vi "Dashboard Main.vi"() -> ()   [LabVIEW 2015]
uses:
  <vilib>/Utility/miscctls.llb/LVRowAndColumnTypeDef.ctl
  <vilib>/event_ctls.llb/eventvkey.ctl
  <vilib>/Rock Robotics/WPI/Dashboard/WPI_DashboardLogging Global.vi
  <vilib>/Rock Robotics/Network Tables/NT Read Boolean.vi
  <vilib>/Rock Robotics/Network Tables/NT Write Numeric Array.vi
  <vilib>/Utility/config.llb/Write Key (String).vi
  <vilib>/Utility/config.llb/Write Key (I32).vi
  <vilib>/Utility/config.llb/NI_LVConfig.lvlib
panel:
  in  "Low Bar":bool
  in  "Cheval":bool
  in  "Portcullis":bool
  in  "Moat":bool
  in  "Ramparts":bool
  in  "R. Terrain":bool
  in  "Rock Wall":bool
  in  "Spy":bool
  in  "Shoot":bool=TRUE
  in  "5":bool
  in  "4":bool
  in  "3":bool
  in  "2":bool
  in  "1":bool
  in  "TCP":refnum<k5>
  in  "Rec Mode":enum32{"Stop", "Record", "Playback"}(radio)
  in  "Vision":u16(ring) items=["Camera Off", "USB Camera SW", "USB Camera HW", "IP Camera"]
  out "Camera IP":string
  out "Image Message":string="Timeout in Camera Communications"
  in  "Dashboard Tab":T1(tab)
  out "Vision\nActive":bool
  out "Level":u8(slide) scale=0.0..3.0
  out "FIRE!!!!":bool
  out "Harvester":dbl
  out "Rotate":dbl
  out "Arm":dbl
  in  "Select Auto":string(combo)
  out "NT Connection":bool
  in  "Camera Settings":T2={"Frame Rate"=30, "Compression"=30, "Size"=1} {"Frame Rate" scale=1.0..30.0; "Size" items=["640x480", "320x240", "160x120"]}
  out "Mode":T3(ring)=enum."Auto Disabled"
  in  "DB Camera Config":bool
  out "fps":dbl format="%#.1g"
  out "Mbps":dbl format="%#.1g"
  out "Mbps LED":bool
  out "Shooter":dbl(knob) scale=0.0..1000.0
  out "Ball Detected":bool
  in  "Custom Auto":bool
  in  "Do Nothing":bool
  in  "File Path":path=path "C:/Users/Rick/Desktop/Robot-2016/autonomous.apple"
  in  "Automode":i32
  out "Error Log":string
  in  "Test Slider":dbl(slide) scale=0.0..100.0 scale format="%#_3g"
  in  "On/Off":bool caption="Solenoid"
  in  "Test Name":u16(ring) items=["Select the test to run..."]
  in  "Test Tree":string(tree)
  in  "Motor":cluster{"Value":dbl, "Enable":bool} {"Value" scale=-1.0..1.0 scale format="%#_3g"}
  out "Progress":T4 {"Test Progress" scale=0.0..100.0}
  in  "Rev/Fwd":cluster{"Forward":bool, "Reverse":bool}
  in  "Test Ring":u16(ring) items=["Monochrome", "Color"]
  out "Cmd Status":string
  in  "Execute Command":bool
  in  "Command Params":string[][](table)
  in  "Command Selection":i32(listbox)
  in  "CheckList":i32(listbox)
  out "Tree":string(tree)
  out "Camera Image":T5(plugin-control)
  out "Background":bool
  # "Batter Shot"
  # "Normal Shot"
  # "Transport"
  # "Harvest"
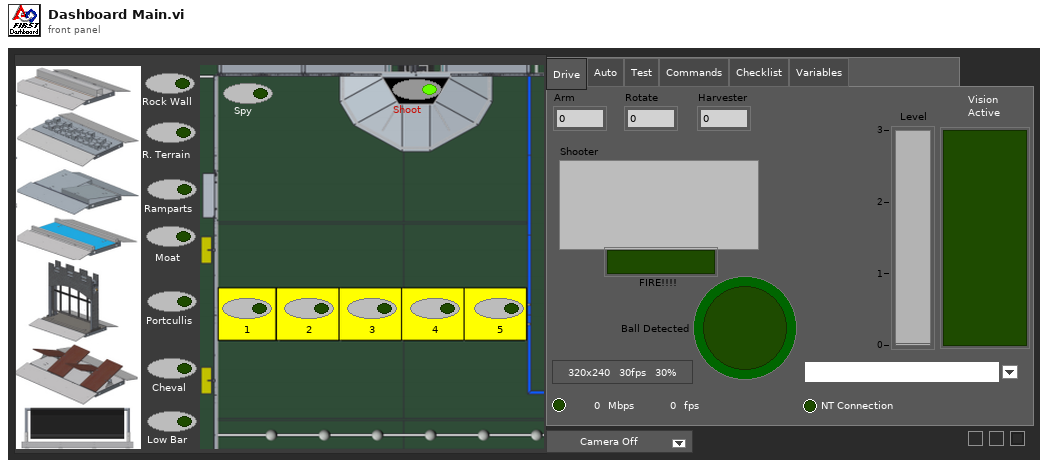
[diagram p1: front panel]
types:
  T1 = enum32{"Drive", "Auto", "Test", "Commands", "Checklist", "Variables"}
  T2 = cluster{"Frame Rate":i32, "Compression":i32, "Size":u16}
  T3 = enum8{"Tele-Op Disabled", "Tele-Op Enabled", "Auto Disabled", "Auto Enabled", "Test Disabled", "Test Enabled", "Disconnected", "No Code", "E-Stop"}
  T4 = cluster{"Test Progress":u8, "Test Progress Text":string}
  T5 = typedef "IMAQ Image.ctl" = refnum<image>
  T6 = cluster{"IDs":cluster{"RPC field ID":u16, "Unique ID":u16}, "String":string}
  T7 = enum32{"Drive", "Basic", "Custom", "Test", "Checklist", "Variables"}
  T8 = typedef "Image Type" = u32
  T9 = cluster{"Camera Image":refnum<vi>, "Dashboard Tab":refnum<vi>, "Background":refnum<vi>, "Vision":refnum<vi>, "Rec Mode":refnum<vi>, "Test Slider":refnum<vi>, "On/Off ":refnum<vi>, "Test Ring":refnum<vi>, "Rev/Fwd":refnum<vi>, "Test Name":refnum<vi>, "Motor":refnum<vi>, "Progress":refnum<vi>, "CheckList":refnum<vi>, "Tree":refnum<vi>, "Test Tree":refnum<vi>, "Command Params":refnum<vi>, "Command Selection":refnum<vi>, "Execute Command":refnum<vi>, "Cmd Status":refnum<vi>}
  T10 = cluster{"Error Strings":string, "Disable Counts":cluster{u16, u16}, "Rail Faults":cluster{u16, u16, u16}, "Robot IP":string, "DB Mode":u8, "Event Info":cluster{"Name":string, "Type":u8, "Number":u16, "Replay":u8}, "Camera Addr":string}
  T11 = cluster{"Storage":cluster{"Disk Free":u64, "RAM Block":u32, "RAM free":u32}, "CPU Utilization":cluster{"CPU % ISR":sgl, "CPU % Time Crit":sgl, "CPU % Timed Str":sgl, "CPU % High":sgl, "CPU % Above":sgl, "CPU % Normal":sgl, "CPU % Low":sgl}, "CAN":cluster{"% Bus Utilization":sgl, "Bus Off Cnt":u32, "TX_FIFO Full Cnt":u32, "Receive Error Cnt":u8, "Transmit Error Cnt":u8}, "HID":cluster{"HID Outputs":u32, "Rumble Low":u16, "Rumble High":u16}[]}
  T12 = cluster{"Status bits":cluster{"Test Mode":bool, "Autonomous":bool, "Enabled":bool, "Code Start":bool, "Brownout":bool, "Reserved 2":bool, "Reserved 3":bool, "E-Stop":bool}, "Code Trace":cluster{"Disabled":bool, "TeleOp":bool, "Auto":bool, "Test":bool}, "Controller Type":enum16{"unknown", "cRIO", "roboRio"}, "Code?":enum16{"unknown", "noCode", "code"}, "Battery V":dbl}
  T13 = cluster{"Control Bits":cluster{"TestMode":bool, "Autonomous":bool, "Enabled":bool, "FMS Present":bool, bool, bool, bool, "E-Stop":bool}, "Team Station ":u8, "Countdown":sgl, "Joystick Values":cluster{"Axes":dbl[], "Buttons":bool[], "POVs":i16[]}[]}
  T14 = typedef "NI_LVConfig.lvlib/Config Data RefNum.ctl" = refnum<k1>
  T15 = cluster{"Operation":enum16{"Update", "Clear"}, "Color Box":u32}[]
  T16 = typedef "eventvkey.ctl" = enum16{"ASCII", "Enter", "Return", "Shift", "Ctrl", "Alt", "Cmd", "Opt", "Caps", "NumLock", "Clear", "Break", "Up", "Down", "Left", "Right", "Insert", "Delete", "Home", "End", "PageUp", "PageDown", "Escape", "Help", "Pause", "ScrollLock", "F1", "F2", "F3", "F4", "F5", "F6", "F7", "F8", "F9", "F10", "F11", "F12", "F13", "F14", "F15", "F16", "F17", "F18", "F19", "F20", "F21", "F22", "F23", "F24", "Play", "VolumeUp", "VolumeDown", "Mute", "Two Byte Char"}
  T17 = cluster{"Image Size":bool, "Image Type":bool, "Pixel Value":bool, "ROI Information":bool, "Zoom Factor":bool}
  T18 = enum8{"Enabled", "Disabled", "Disabled and Grayed Out"}
  T19 = cluster{"Operation":enum16{"Update", "Clear"}, "Color Box":u32}
  T20 = typedef "LVRowAndColumnTypeDef.ctl" = cluster{"Row":i32, "Column":i32}
  T21 = cluster{"Shift":bool, "Ctrl":bool, "Alt":bool, "Cmd":bool, "Opt":bool}
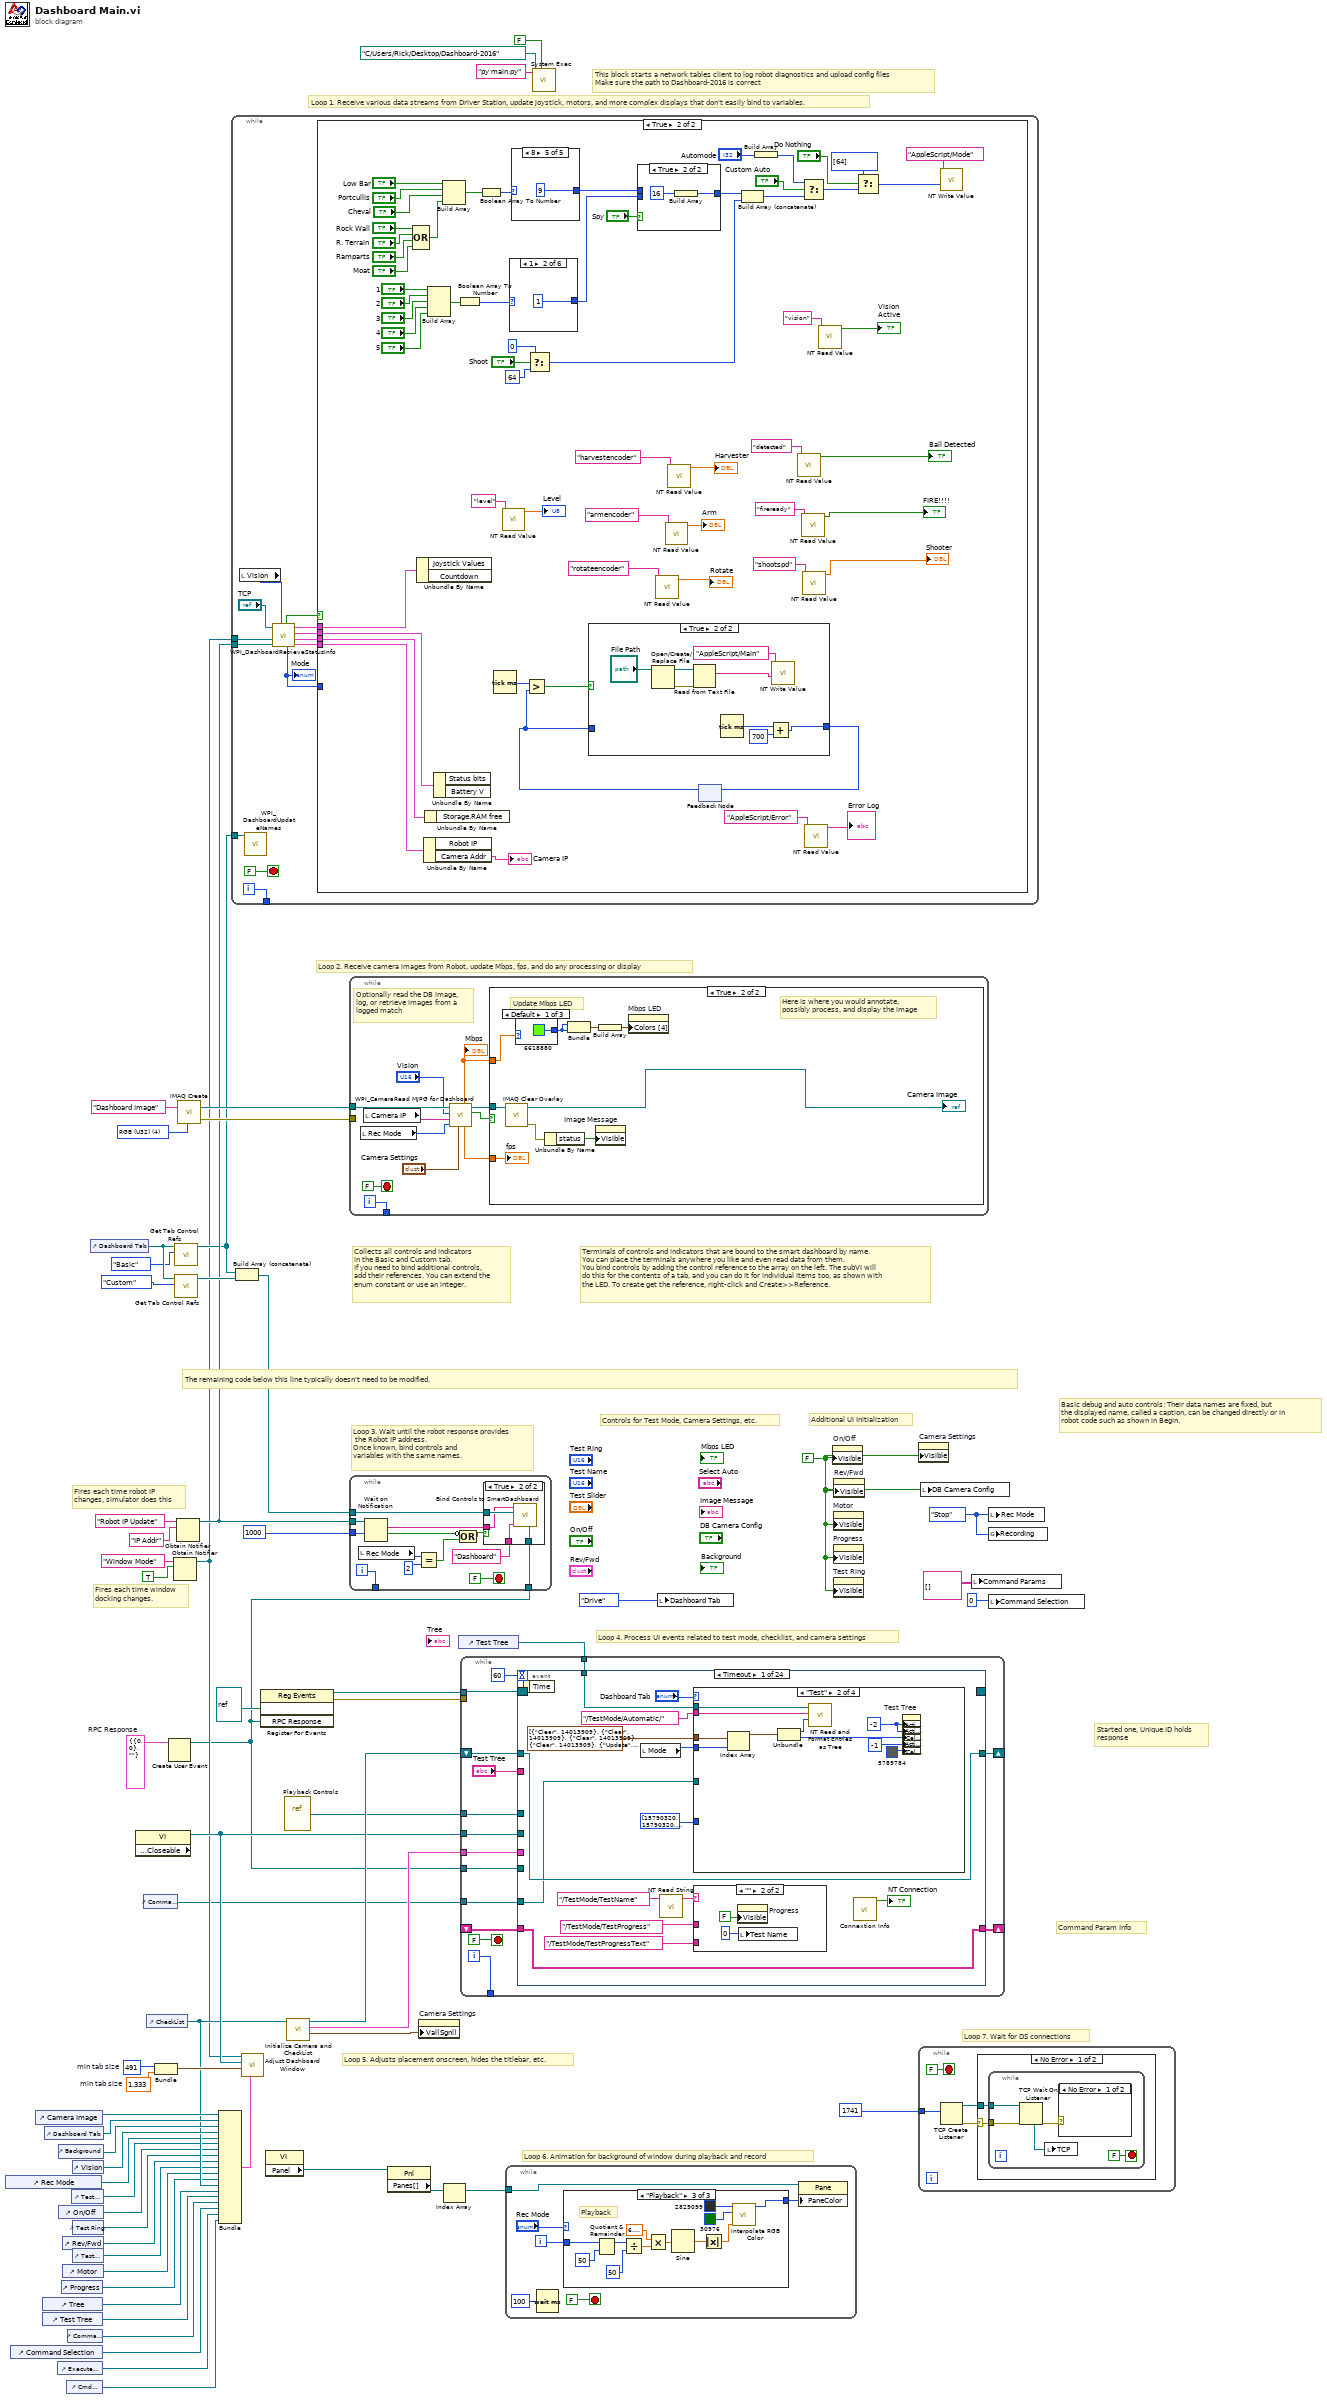
[diagram p0: block diagram]
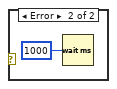
[diagram p2: hidden frame]
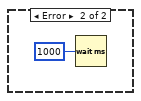
[diagram p3: hidden frame]
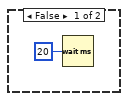
[diagram p4: hidden frame]
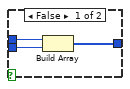
[diagram p5: hidden frame]
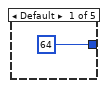
[diagram p6: hidden frame]
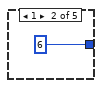
[diagram p7: hidden frame]
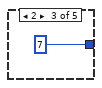
[diagram p8: hidden frame]
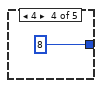
[diagram p9: hidden frame]
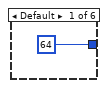
[diagram p10: hidden frame]
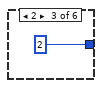
[diagram p11: hidden frame]
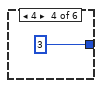
[diagram p12: hidden frame]
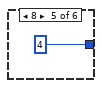
[diagram p13: hidden frame]
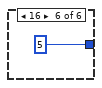
[diagram p14: hidden frame]
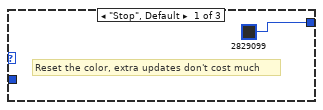
[diagram p16: hidden frame]
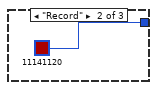
[diagram p17: hidden frame]
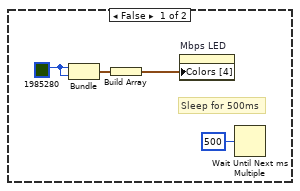
[diagram p19: hidden frame]
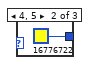
[diagram p20: hidden frame]
diagram:
  w11 = T6 {"IDs"={"RPC field ID"=0, "Unique ID"=0}, "String"=""}  # RPC Response
  w36 = 491  # min tab size
  w35 = 1.333  # min tab size
  w44 = enum32{"Stop", "Record", "Playback"}."Stop" ("Rec Mode")
  w18 = FALSE ("Visible")
  w64 = T8 4 items=["Grayscale (U8)", "Grayscale (I16)", "Grayscale (SGL)", "Complex (CSG)", "RGB (U32)", "HSL (U32)", "RGB (U64)"] ("Image Type")
  # "This block starts a network tables client to log robot diagnostics and upload config files\nMake sure the path to Dashboard-2016 is correct"
  # "Command Param Info"
  # "Started one, Unique ID holds\nresponse"
  # "Loop 7. Wait for DS connections"
  # "Basic debug and auto controls: Their data names are fixed, but\nthe displayed name, called a caption, can be changed directly or in\nrobot code such as shown in Begin."
  # "Controls for Test Mode, Camera Settings, etc."
  # "Additional UI Initialization"
  # "Loop 6. Animation for background of window during playback and record"
  # "Fires each time robot IP\nchanges, simulator does this"
  # "Fires each time window\ndocking changes."
  # "Collects all controls and indicators\nin the Basic and Custom tab.\nIf you need to bind additional controls,\nadd their references. You can extend the\nenum constant or use an integer."
  # "The remaining code below this line typically doesn't need to be modified."
  # "Loop 4. Process UI events related to test mode, checklist, and camera settings"
  # "Terminals of controls and indicators that are bound to the smart dashboard by name.\nYou can place the terminals anywhere you like and even read data from them.\nYou bind controls by adding the control reference to the array on the left. The subVI will\ndo this for the contents of a tab, and you can do it for individual items too, as shown with\nthe LED. To create get the reference, right-click and Create>>Reference."
  # "Loop 3. Wait until the robot response provides\n the Robot IP address.\nOnce known, bind controls and\nvariables with the same names."
  # "Loop 5. Adjusts placement onscreen, hides the titlebar, etc."
  # "Loop 1. Receive various data streams from Driver Station, update joystick, motors, and more complex displays that don't easily bind to variables."
  # "Loop 2. Receive camera images from Robot, update Mbps, fps, and do any processing or display"
  n1 = control-ref of="Rec Mode"() -> (w24:refnum<vi>)
  n2 = control-ref of="Command Selection"() -> (w10:refnum<vi>)
  n3 = control-ref of="Camera Image"() -> (w39:refnum<vi>)
  n4 = control-ref of="Tree"() -> (w28:refnum<vi>)
  n5 = control-ref of="Test Tree"() -> (w27:refnum<vi>)
  n6 = control-ref of="Dashboard Tab"() -> (w38:refnum<vi>)
  n7 = control-ref of="Execute Command"() -> (w12:refnum<vi>)
  n8 = control-ref of="Background"() -> (w33:refnum<vi>)
  n9 = control-ref of="On/Off"() -> (w22:refnum<vi>)
  n10 = control-ref of="Progress"() -> (w19:refnum<vi>)
  n11 = control-ref of="Rev/Fwd"() -> (w20:refnum<vi>)
  n12 = control-ref of="Motor"() -> (w25:refnum<vi>)
  n13 = control-ref of="Cmd Status"() -> (w6:refnum<vi>)
  n14 = control-ref of="Command Params"() -> (w13:refnum<vi>)
  n15 = control-ref of="Test Slider"() -> (w23:refnum<vi>)
  n16 = control-ref of="Vision"() -> (w37:refnum<vi>)
  n17 = control-ref of="Test Ring"() -> (w21:refnum<vi>)
  n18 = control-ref of="Test Name"() -> (w26:refnum<vi>)
  n19 = control-ref of="Dashboard Tab"() -> (w42:refnum<vi>)
  n20 = property class="VI" props=["Front Panel.Closeable"]() -> (reference out=w43:refnum<vi>)  [unwired: 2 in, 2 out]
  n21 = control-ref of="Command Params"() -> (w5:refnum<vi>)
  n22 = control-ref of="CheckList"() -> (w29:refnum<vi>)
  n23 = Bundle("min tab size"=w36, "min tab size"=w35) -> (w34:cluster{"min tab size":i32, "min tab size":dbl})  [unwired: 1 in]
  n24 = Create User Event(user event datatype=w11) -> (user event=w7:refnum<user-event>)  [unwired: 1 in, 1 out]
  n25 = Obtain Notifier(name (unnamed)="Window Mode", notification data type=TRUE) -> (notifier out=w15:refnum<notifier>)  [unwired: 2 in, 2 out]
  n26 = call <vilib>:"Get Tab Control Refs.vi"("Page Index"=T7."Basic" ("Dashboard Tab"), "TabControl in"=w42) -> ("ControlsOnPage"=w16:refnum<vi>[])  [unwired: 9 in]
  n27 = call <vilib>:"Get Tab Control Refs.vi"("Page Index"=T7."Custom" ("Dashboard Tab"), "TabControl in"=w42) -> ("ControlsOnPage"=w41:refnum<vi>[])  [unwired: 9 in]
  n28 = Obtain Notifier(name (unnamed)="Robot IP Update", notification data type="IP Addr" ("name (unnamed)")) -> (notifier out=w17:refnum<notifier>)  [unwired: 2 in, 2 out]
  n29 = call "IMAQ Create"("Image Name"="Dashboard Image", "Image Type"=w64) -> ("New Image"=w62:T5, "error out"=w61:errorcluster)  [unwired: 2 in, 1 out]
  n30 = Bundle("Camera Image"=w39, "Dashboard Tab"=w38, "Background"=w33, "Vision"=w37, "Rec Mode"=w24, "Test Slider"=w23, "On/Off"=w22, "Test Ring"=w21, "Rev/Fwd"=w20, "Test Name"=w26, "Motor"=w25, "Progress"=w19, "CheckList"=w29, "Tree"=w28, "Test Tree"=w27, "Command Params"=w13, "Command Selection"=w10, "Execute Command"=w12, "Cmd Status"=w6) -> (w30:T9)  [unwired: 1 in]
  n31 = while {
    tunnel: [w76] -> _
    tunnel: w17 -> [w70]
    tunnel: w16 -> [w69]
    tunnel: w15 -> [w65]
    i -> [w76]
    stop <- FALSE stop-if-true
    n32 = local read "Vision"() -> (w67:u16)
    n33 = call <vilib>:"WPI_DashboardUpdateNames.vi"("Controls on Tab"=w69) -> ()  [unwired: 11 in]
    n34 = call <vilib>:"WPI_DashboardRetrieveStatusInfo.vi"("Vision"=w67, "Binding Refnum"=w70, "Window Mode Notifier"=w65, "TCP Cnx"="TCP") -> ("Power and Errors"=w71:T10, "Robot Metrics"=w74:T11, "Status Info"=w75:T12, "Control Info"=w72:T13, "Robot Mode"=w68:T3, "Process?"=w73:bool)  [unwired: 2 in]
    "Mode" <- w68
    n35 = case shown="True" w73 {
      tunnel: w75 -> [_ w139]
      tunnel: w74 -> [_ w138]
      tunnel: w72 -> [_ w137]
      tunnel: w71 -> [_ w136]
      tunnel: w68 -> [_ _]
      frame False {
        n36 = Wait (ms)(milliseconds to wait=u32 20) -> ()  [unwired: 1 out]
      }
      frame True {
        n37 = Compound Arithmetic op=OR("Rock Wall", "R. Terrain", "Ramparts", "Moat") -> (w98:bool)
        n38 = Unbundle By Name(w137) -> ()  [unwired: 2 out]
        n39 = Unbundle By Name(w136) -> ("Camera Addr"=→"Camera IP":string)  [unwired: 1 out]
        n40 = Unbundle By Name(w138) -> ()  [unwired: 1 out]
        n41 = Build Array("1", "2", "3", "4", "5") -> (w108:bool[])
        n42 = Unbundle By Name(w139) -> ()  [unwired: 2 out]
        n43 = Build Array("Low Bar", "Portcullis", "Cheval", w98) -> (w97:bool[])
        n44 = Boolean Array To Number(Boolean array=w108) -> (number=w107:u32)
        n45 = Boolean Array To Number(Boolean array=w97) -> (number=w106:u32)
        n46 = Tick Count (ms)() -> (millisecond timer value=w133:u32)
        n47 = call-poly <vilib>:"NT Read Value.vi"("Name"="level") -> ("Numeric"=→"Level":dbl)  [unwired: 9 in, 1 out]
        n48 = case shown="1" w107 {
          tunnel: [64 1 2 3 4 5] -> w95
          frame Default {
          }
          frame 1 {
          }
          frame 2 {
          }
          frame 4 {
          }
          frame 8 {
          }
          frame 16 {
          }
        }
        n49 = case shown="8" w106 {
          tunnel: [64 6 7 8 9] -> w96
          frame Default {
          }
          frame 1 {
          }
          frame 2 {
          }
          frame 4 {
          }
          frame 8 {
          }
        }
        n50 = Select(t=0, s="Shoot", f=64) -> (s? t:f=w89:i32)
        n51 = case shown="True" "Spy" {
          tunnel: w96 -> [w142 _]
          tunnel: w95 -> [w141 _]
          tunnel: [w140 w143] -> w90
          frame False {
            n52 = Build Array(w142, w141) -> (w140:i32[])
          }
          frame True {
            n53 = Build Array(16) -> (w143:i32[])
          }
        }
        n54 = call-poly <vilib>:"NT Read Value.vi"("Name"="rotateencoder") -> ("Numeric"=→"Rotate":dbl)  [unwired: 9 in, 1 out]
        n55 = call-poly <vilib>:"NT Read Value.vi"("Name"="armencoder") -> ("Numeric"=→"Arm":dbl)  [unwired: 9 in, 1 out]
        n56 = call-poly <vilib>:"NT Read Value.vi"("Name"="harvestencoder") -> ("Numeric"=→"Harvester":dbl)  [unwired: 9 in, 1 out]
        n57 = feedback #1() -> (w132:u32)  [unwired: 1 in]
        n58 = Greater?(x=w133, y=w132) -> (0:w131:bool)
        n59 = case shown="True" w131 {
          tunnel: w132 -> [w156 _]
          tunnel: [w156 w160] -> w134
          frame False {
          }
          frame True {
            n60 = Open/Create/Replace File(file path (use dialog)="File Path") -> (refnum out=w163:refnum<file>, error out=w164:errorcluster)  [unwired: 5 in, 1 out]
            n61 = Read from Text File(file (use dialog)=w163, error in=w164) -> (text=w158:string)  [unwired: 2 in, 3 out]
            n62 = Tick Count (ms)() -> (millisecond timer value=w161:u32)
            n63 = Add(x=w161, y=u32 700) -> (x+y=w160:u32)
            n64 = call-poly <vilib>:"NT Write Value.vi"("String"=w158, "Name"="AppleScript/Main") -> ()  [unwired: 9 in, 1 out]
          }
        }
        n65 = feedback-in #1(w134) -> ()
        n66 = Build Array (concatenate)(w90, w89) -> (w88:i32[])
        n67 = Build Array("Automode") -> (w85:i32[])
        n68 = call-poly <vilib>:"NT Read Value.vi"("Name"="detected") -> ("Boolean"=→"Ball Detected":bool)  [unwired: 9 in, 1 out]
        n69 = call-poly <vilib>:"NT Read Value.vi"("Name"="fireready") -> ("Boolean"=→"FIRE!!!!":bool)  [unwired: 9 in, 1 out]
        n70 = Select(t=w85, s="Custom Auto", f=w88) -> (s? t:f=w84:i32[])
        n71 = call-poly <vilib>:"NT Read Value.vi"("Name"="shootspd") -> ("Numeric"=→"Shooter":dbl)  [unwired: 9 in, 1 out]
        n72 = call-poly <vilib>:"NT Read Value.vi"("Name"="AppleScript/Error") -> ("String"=→"Error Log":string)  [unwired: 9 in, 1 out]
        n73 = call-poly <vilib>:"NT Read Value.vi"("Name"="vision") -> ("Boolean"=→"Vision\nActive":bool)  [unwired: 9 in, 1 out]
        n74 = Select(t=i32[] [64], s="Do Nothing", f=w84) -> (s? t:f=w81:i32[])
        n75 = call-poly <vilib>:"NT Write Value.vi"("Numeric Array"=w81, "Name"="AppleScript/Mode") -> ()  [unwired: 9 in, 1 out]
      }
    }
  }
  n76 = Build Array (concatenate)(w16, w41) -> (w40:refnum<vi>[])
  n77 = call "Adjust Dashboard Window.vi"("Sizing Refnums"=w30, "Size Constraints"=w34, "VI"=w43, "WIn Mode"=w15) -> ()  [unwired: 8 in]
  n78 = register-events(refnum<vi> refnum, w7) -> (reference out=w48:refnum<event-registration>, error out=w47:errorcluster)  [unwired: 2 in]
  n79 = property class="VI"() -> ("Panel"=w51:refnum<vi>)  [unwired: 2 in, 2 out]
  n80 = vi-ref "Playback Controls.vi"() -> (w49:refnum<vi>)
  n81 = call "Initialize Camera and CheckList.vi"("ListBox in"=w29) -> ("Cluster"=w55:cluster{"value":i32, "value":i32, "index":i32}, "Array"=w56:cluster{string[]}[], "File Refnum"=w54:T14)  [unwired: 8 in]
  n82 = while {
    tunnel: w62 -> [w173]
    tunnel: w61 -> [_]
    tunnel: [w174] -> _
    i -> [w174]
    stop <- FALSE stop-if-true
    # "Optionally read the DB image,\nlog, or retrieve images from a\nlogged match"
    n83 = local read "Rec Mode"() -> (w168:enum32{"Stop", "Record", "Playback"})
    n84 = local read "Camera IP"() -> (w166:string)
    n85 = call <vilib>:"WPI_CameraRead MJPG for Dashboard.vi"("Camera Settings"="Camera Settings", "Rec Mode"=w168, "Camera IP"=w166, "Camera Mode"="Vision", "Refnum in"=w173) -> ("Active"=w171:bool, "Refnum out"=w172:T5, "FPS"=w170:dbl, "Bandwidth (Mbps)"=w165:dbl)  [unwired: 3 in]
    "Mbps" <- w165
    n86 = case shown="True" w171 {
      tunnel: w172 -> [_ w183]
      tunnel: w165 -> [_ w182]
      tunnel: w170 -> [_ w181]
      frame False {
        w176 = u32 1985280 ("Color Box")
        # "Sleep for 500ms"
        n87 = Bundle("Color Box"=w176, "Color Box"=w176) -> (w178:cluster{"Color Box":u32, "Color Box":u32})  [unwired: 1 out]
        n88 = Build Array(w178) -> (w177:cluster{"Color Box":u32, "Color Box":u32}[])
        n89 = property on="Mbps LED" class="Bool (strict)"("Colors [4]"=w177) -> ()  [unwired: 2 in, 2 out]
        n90 = Wait Until Next ms Multiple(millisecond multiple=u32 500) -> ()  [unwired: 1 out]
      }
      frame True {
        # "Here is where you would annotate,\npossibly process, and display the image"
        # "Update Mbps LED"
        n91 = call "IMAQ Clear Overlay"("Image"=w183) -> ("error out"=w187:errorcluster, "Image Out"=→"Camera Image":T5)  [unwired: 2 in, 7 out]
        n92 = case shown="Default" w182 {
          tunnel: [u32 6618880 ("Color Box") u32 16776722 ("Color Box") u32 16716800 ("Color Box")] -> w184
          frame Default {
          }
          frame 4, 5 {
          }
          frame 6.. {
          }
        }
        n93 = Unbundle By Name(w187) -> ("status"=w188:bool)
        n94 = Bundle("Color Box"=w184, "Color Box"=w184) -> (w186:cluster{"Color Box":u32, "Color Box":u32})  [unwired: 1 out]
        n95 = property on="Image Message" class="Str"("Visible"=w188) -> ()  [unwired: 2 in, 2 out]
        n96 = Build Array(w186) -> (w185:cluster{"Color Box":u32, "Color Box":u32}[])
        n97 = property on="Mbps LED" class="Bool (strict)"("Colors [4]"=w185) -> ()  [unwired: 2 in, 2 out]
        "fps" <- w181
      }
    }
  }
  n98 = while {
    tunnel: w40 -> [w204]
    tunnel: w17 -> [w202]
    tunnel: [w200] -> _
    tunnel: u32 1000 ("milliseconds to wait") -> [w199]
    tunnel: w7 -> [w192]
    i -> [w200]
    stop <- FALSE stop-if-true
    n99 = local read "Rec Mode"() -> (w195:enum32{"Stop", "Record", "Playback"})
    n100 = Wait on Notification(notifier=w202, timeout in ms (-1)=w199) -> (notification=w201:string, timed out?=w197:bool)  [unwired: 2 in, 2 out]
    n101 = Equal?(x=w195, y=u16 2 ("Rec Mode")) -> (x = y?=w196:bool)
    n102 = Compound Arithmetic op=OR(invert w197, w196) -> (w198:bool)
    n103 = case shown="True" w198 {
      tunnel: w204 -> [_ w208]
      tunnel: w201 -> [_ w207]
      tunnel: "Dashboard" -> [_ w206]
      tunnel: w192 -> [_ w205]
      frame False {
      }
      frame True {
        n104 = call <vilib>:"Bind Controls to SmartDashboard.vi"("RPC ref"=w205, "Client Name"=w206, "Bound Control Refs"=w208, "Server IP Address"=w207) -> ()  [unwired: 8 in]
      }
    }
  }
  n105 = property class="Pnl"(reference=w51) -> ("Panes[]"=w52:refnum<vi>[])  [unwired: 1 in, 2 out]
  n106 = property on="Camera Settings" class="Clust (strict)"("Val(Sgnl)"=w55) -> ()  [unwired: 2 in, 2 out]
  n107 = Index Array(array=w52) -> (element=w50:refnum<vi>)  [unwired: 1 in]
  n108 = control-ref of="Test Tree"() -> (w53:refnum<vi>)
  n109 = while {
    tunnel: w56 -> [w220]
    shift-right: [w219] -> _
    shift-left: w54 -> [w218]
    tunnel: [w217] -> _
    tunnel: w53 -> [w216]
    tunnel: w49 -> [w215]
    tunnel: w48 -> [w214]
    tunnel: w47 -> [_]
    tunnel: w43 -> [w213]
    tunnel: w7 -> [w212]
    tunnel: w5 -> [w211]
    shift-right: [w210] -> _
    shift-left: _ -> [w209]
    i -> [w217]
    stop <- FALSE stop-if-true
    n110 = event shown="[0] Timeout" {
      selector: w214 -> [_ _ _ _ _ _ _ _ _ _ _ _ _ _ _ _ _ _ _ _ _ _ _ _]
      dyn-events: [_ _ _ _ _ _ _ _ _ _ _ _ _ _ _ _ _ _ w529 _ _ _ _ _] -> _
      timeout: u32 60 ("milliseconds to wait") -> [_ _ _ _ _ _ _ _ _ _ _ _ _ _ _ _ _ _ _ _ _ _ _ _]
      tunnel: w216 -> [w233 _ _ _ _ _ _ _ _ _ _ _ _ _ _ _ _ _ _ _ _ _ _ _]
      tunnel: "Test Tree" -> [_ _ _ _ _ _ _ _ _ _ _ _ _ w492 w501 w504 w509 w518 _ _ _ _ _ _]
      tunnel: w220 -> [_ w271 _ _ _ _ _ _ _ _ _ w454 w485 _ _ _ _ _ _ _ _ _ _ _]
      tunnel: [w230 w270 w374 w380 w390 w394 w400 w412 w420 w426 w439 w453 w478 w491 w499 w503 w508 w517 w531 w547 w549 w557 w568 w573] -> w219
      tunnel: w218 -> [w230 w270 w374 w380 w390 w394 w400 w412 w420 w426 w439 w452 w478 w491 w499 w503 w508 w517 w531 w547 w549 w557 w568 w573]
      tunnel: w215 -> [_ _ _ _ _ _ _ _ _ _ _ _ _ _ _ _ _ _ w532 _ w552 _ _ _]
      tunnel: w213 -> [_ _ _ _ _ _ _ _ _ _ _ _ _ _ _ _ _ _ w527 _ _ _ _ _]
      tunnel: w212 -> [_ _ _ _ _ _ _ _ _ _ _ _ _ _ _ _ _ _ w523 _ _ _ _ _]
      tunnel: w211 -> [w225 _ _ _ _ _ w398 _ _ _ _ _ _ _ _ _ _ _ _ _ _ _ _ _]
      tunnel: [w224 w269 w373 w379 w389 w395 w396 w406 w417 w425 w438 w451 w477 w490 w498 w502 w507 w516 w522 w545 w548 w553 w561 w574] -> w210
      tunnel: w209 -> [w224 w269 w373 w379 w389 w395 w396 _ _ w425 w438 w451 w477 w490 w498 w502 w507 w516 w522 w545 w548 w553 w561 w574]
      event Timeout {
        n111 = event-data() -> ()  [unwired: 1 in, 1 out]
        n112 = local read "Mode"() -> (w227:T3)
        n113 = call <vilib>:"NT Read String.vi"("Name"="/TestMode/TestName") -> ("String"=w236:string)  [unwired: 9 in, 1 out]
        n114 = case shown="\"Test\"" "Dashboard Tab" {
          tunnel: w233 -> [_ w247 _ _]
          tunnel: "/TestMode/Automatic/" ("Name Pattern") -> [_ w246 _ _]
          tunnel: T15 [{"Operation"=enum."Clear", "Color Box"=14013909}, {"Operation"=enum."Clear", "Color Box"=14013909}, {"Operation"=enum."Clear", "Color Box"=14013909}, {"Operation"=enum."Clear", "Color Box"=14013909}, {"Operation"=enum."Update", "Color Box"=14013909}, {"Operation"=enum."Update", "Color Box"=16777215}, {"Operation"=enum."Clear", "Color Box"=14013909}, {"Operation"=enum."Clear", "Color Box"=14013909}, {"Operation"=enum."Clear", "Color Box"=14013909}] -> [_ w239 _ w256]
          tunnel: w227 -> [_ w238 _ w255]
          tunnel: u32[] [15790320, 15790320, 15790320, 15790320, 16777215, 16777215, 15790320, 15790320, 15790320] -> [_ _ _ w261]
          tunnel: w225 -> [_ _ _ w249]
          frame "Auto", Default {
          }
          frame "Test" {
            w245 = -2 ("Active Item:Row Number")
            n115 = Index Array(array=w239, index=w238) -> (element=w240:T19)
            n116 = Unbundle(w240) -> ("Operation"=w241:enum16{"Update", "Clear"}, "Color Box"=w242:u32)
            n117 = call <vilib>:"NT Read and Format Entries as Tree.vi"("Operation"=w241, "Name Pattern"=w246, "Tree Refnum"=w247) -> ()  [unwired: 7 in, 2 out]
            n118 = property on="Test Tree" class="Tree (strict)"("Active Item Row Number"=w245, "ActiveColNum"=w245, "CellBG"=w242, "Active Item Row Number"=-1 ("Active Item:Row Number"), "CellBG"=u32 5789784 ("Color Box")) -> ()  [unwired: 2 in, 2 out]
          }
          frame "Variables" {
            n119 = control-ref of="Tree"() -> (w248:refnum<vi>)
            n120 = call <vilib>:"NT Read and Format Entries as Tree.vi"("Tree Refnum"=w248) -> ()  [unwired: 9 in, 2 out]
          }
          frame "Commands" {
            w257 = u32 5789784 ("Color Box")
            w258 = T20 {"Row"=-1, "Column"=-2} ("Active Cell:Active Cell")
            w260 = T20 {"Row"=-2, "Column"=-2} ("Active Cell:Active Cell")
            n121 = Index Array(array=w261, index=w255) -> (element=w259:u32)
            n122 = Index Array(array=w256, index=w255) -> (element=w254:T19)
            n123 = Unbundle(w254) -> ("Operation"=w253:enum16{"Update", "Clear"})  [unwired: 1 out]
            n124 = local read "Command Selection"() -> (w252:i32)
            n125 = property on="Command Selection" class="MCListbox (strict)"("ActiveCell"=w260, "CellBG"=w259, "ActiveCell"=w258, "CellBG"=w257) -> ()  [unwired: 2 in, 2 out]
            n126 = call <vilib>:"WPI_DashboardUpdate RPC Info.vi"("Operation"=w253) -> ("update"=w251:bool, "commands"=w250:string[][])  [unwired: 9 in]
            n127 = property on="Command Selection" class="MCListbox (strict)"("ItemNames"=w250) -> ()  [unwired: 2 in, 2 out]
            n128 = property on="Command Params" class="Tbl (strict)"("Active Cell"=w260, "Cell BG Color"=w259, "Active Cell"=w258, "Cell BG Color"=w257) -> ()  [unwired: 2 in, 2 out]
            n129 = call <vilib>:"WPI_DashboardUpdate Command Params.vi"("Update"=w251, "NewVal"=w252, "Commands"=w250, "Param Tbl"=w249) -> ()  [unwired: 7 in, 1 out]
          }
        }
        n130 = case shown="\"\"" w236 {
          tunnel: "/TestMode/TestProgress" ("Name") -> [w263 _]
          tunnel: "/TestMode/TestProgressText" ("Name") -> [w262 _]
          frame Default {
            n131 = call <vilib>:"NT Read Number.vi"("Name"=w263) -> ("Numeric"=w264:dbl)  [unwired: 9 in, 1 out]
            n132 = call <vilib>:"NT Read String.vi"("Name"=w262) -> ("String"=w265:string)  [unwired: 9 in, 1 out]
            n133 = Bundle("Numeric"=w264, "String"=w265) -> (→"Progress":cluster{"Numeric":dbl, "String":string})  [unwired: 1 in]
          }
          frame "" {
            n134 = property on="Progress" class="Clust (strict)"("Visible"=FALSE) -> ()  [unwired: 2 in, 2 out]
            n135 = local write "Test Name"(u16 0) -> ()
          }
        }
        n136 = call <vilib>:"Connextion Info.vi"() -> ("Connected"=→"NT Connection":bool)  [unwired: 10 in, 1 out]
      }
      event "Test Tree": Value Change {
        # "Show appropriate\ncontrols"
        n137 = event-data() -> ("CtlRef"=w274:refnum<vi>, "NewVal"=w272:string)  [unwired: 1 in]
        n138 = call <vilib>:"WPI_UtilitiesGetTreeIOName.vi"("NewVal"=w272, "TreeControl in"=w274) -> ("I/O Name"=w275:string)  [unwired: 9 in]
        n139 = case shown="\"Analog Out\", \"Motor\", \"PWM\"" w275 {
          selector: w275 -> [_ w282 _ w304 w313 _]
          tunnel: w272 -> [_ _ w301 w303 _ w320]
          tunnel: w271 -> [_ _ _ _ _ w319]
          frame Default {
            w277 = FALSE ("Visible")
            w276 = FALSE ("Visible")
            n140 = property on="Motor" class="Clust (strict)"("Visible"=w276) -> ()  [unwired: 2 in, 2 out]
            n141 = property on="Test Ring" class="Ring (strict)"("Visible"=w276) -> ()  [unwired: 2 in, 2 out]
            n142 = property on="Rev/Fwd" class="Clust (strict)"("Visible"=w277) -> ()  [unwired: 2 in, 2 out]
            n143 = property on="On/Off" class="Bool (strict)"("Visible"=w277) -> ()  [unwired: 2 in, 2 out]
            n144 = property on="Test Slider" class="Slide (strict)"("Visible"=w277) -> ()  [unwired: 2 in, 2 out]
          }
          frame "Analog Out", "Motor", "PWM" {
            w283 = FALSE ("Visible")
            n145 = case shown="\"Analog Out\"" w282 {
              tunnel: [1.0 ("Value") -1.0 ("Value") 0.0 ("Value")] -> w281
              tunnel: [255.0 ("Value") 1.0 ("Value") 5.0 ("Value")] -> w280
              tunnel: [128.0 ("Value") 0.0 ("Value") 0.0 ("Value")] -> w279
              tunnel: [64.0 ("Value") 0.5 ("Value") 1.0 ("Value")] -> w278
              frame "PWM" {
              }
              frame "Motor", Default {
              }
              frame "Analog Out" {
              }
            }
            n146 = property on="Motor" class="Clust (strict)"("Visible"=TRUE) -> ()  [unwired: 2 in, 2 out]
            n147 = property on="Value" class="Slide (strict)"("Value"=w279, "Scale.Minimum"=w281, "Scale.Maximum"=w280, "Scale.Increment"=w278) -> ()  [unwired: 2 in, 2 out]
            n148 = property on="On/Off" class="Bool (strict)"("Visible"=w283) -> ()  [unwired: 2 in, 2 out]
            n149 = property on="Test Slider" class="Slide (strict)"("Visible"=w283) -> ()  [unwired: 2 in, 2 out]
            n150 = property on="Test Ring" class="Ring (strict)"("Visible"=w283) -> ()  [unwired: 2 in, 2 out]
            n151 = property on="Rev/Fwd" class="Clust (strict)"("Visible"=w283) -> ()  [unwired: 2 in, 2 out]
          }
          frame "Servo" {
            w299 = FALSE ("Visible")
            n152 = call <vilib>:"NT Read Number.vi"("Name"=w301) -> ("Numeric"=w300:dbl)  [unwired: 9 in, 1 out]
            n153 = property on="Test Slider" class="Slide (strict)"("Visible"=TRUE, "Scale.Maximum"=170.0 ("Scale.Range:Maximum")) -> ()  [unwired: 2 in, 2 out]
            n154 = local write "Test Slider"(w300) -> ()
            n155 = property on="Motor" class="Clust (strict)"("Visible"=w299) -> ()  [unwired: 2 in, 2 out]
            n156 = property on="Rev/Fwd" class="Clust (strict)"("Visible"=w299) -> ()  [unwired: 2 in, 2 out]
            n157 = property on="On/Off" class="Bool (strict)"("Visible"=w299) -> ()  [unwired: 2 in, 2 out]
            n158 = property on="Test Ring" class="Ring (strict)"("Visible"=w299) -> ()  [unwired: 2 in, 2 out]
          }
          frame "Relay", "Solenoid" {
            w302 = FALSE ("Visible")
            n159 = property on="Motor" class="Clust (strict)"("Visible"=w302) -> ()  [unwired: 2 in, 2 out]
            n160 = property on="Test Slider" class="Slide (strict)"("Visible"=w302) -> ()  [unwired: 2 in, 2 out]
            n161 = Search and Replace String(input string=w303, search string="/Value  **", replace string="/Direction") -> (result string=w309:string)  [unwired: 5 in, 3 out]
            n162 = property on="Test Ring" class="Ring (strict)"("Visible"=w302) -> ()  [unwired: 2 in, 2 out]
            n163 = call <vilib>:"NT Read String.vi"("Name"=w309) -> ("String"=w307:string)  [unwired: 9 in, 1 out]
            n164 = Equal?(x="Both directions", y=w307) -> (x = y?=w305:bool)
            n165 = Not(x=w305) -> (.not. x?=w306:bool)
            n166 = property on="Rev/Fwd" class="Clust (strict)"("Visible"=w305) -> ()  [unwired: 2 in, 2 out]
            n167 = property on="On/Off" class="Bool (strict)"("Visible"=w306, "Caption.Text"=w304) -> ()  [unwired: 2 in, 2 out]
          }
          frame "Compressor", "Digital Out" {
            w312 = FALSE ("Visible")
            # "Get direction and finish"
            n168 = property on="Motor" class="Clust (strict)"("Visible"=w312) -> ()  [unwired: 2 in, 2 out]
            n169 = property on="Test Slider" class="Slide (strict)"("Visible"=w312) -> ()  [unwired: 2 in, 2 out]
            n170 = property on="Test Ring" class="Ring (strict)"("Visible"=w312) -> ()  [unwired: 2 in, 2 out]
            n171 = property on="On/Off" class="Bool (strict)"("Visible"=TRUE, "Caption.Text"=w313) -> ()  [unwired: 2 in, 2 out]
            n172 = property on="Rev/Fwd" class="Clust (strict)"("Visible"=FALSE) -> ()  [unwired: 2 in, 2 out]
          }
          frame "Camera" {
            n173 = call <vilib>:"Get Last Path Segment.vi"("String in"=w320) -> ("String out"=w321:string)  [unwired: 10 in]
            n174 = property on="On/Off" class="Bool (strict)"("Visible"=FALSE) -> ()  [unwired: 2 in, 2 out]
            n175 = property on="Motor" class="Clust (strict)"("Visible"=FALSE) -> ()  [unwired: 2 in, 2 out]
            n176 = property on="Rev/Fwd" class="Clust (strict)"("Visible"=FALSE) -> ()  [unwired: 2 in, 2 out]
            n177 = case shown="\"White Balance  **\"" w321 {
              tunnel: w320 -> [w327 w336 w345 w354 w363 _ w369]
              tunnel: w319 -> [w325 w333 w342 w351 w360 _ _]
              frame "Size  **" {
                n178 = Index Array(array=w325) -> (element=w324:cluster{string[]})  [unwired: 1 in]
                n179 = call <vilib>:"NT Read String.vi"("Name"=w327) -> ("String"=w326:string)  [unwired: 9 in, 1 out]
                n180 = Unbundle(w324) -> (w322:string[])
                n181 = Match First String(2:w322, 3:w326) -> (0:w323:i32)  [unwired: 1 out]
                n182 = property on="Test Ring" class="Ring (strict)"("Value"=w323, "Strings []"=w322) -> ()  [unwired: 2 in, 2 out]
                n183 = property on="Test Ring" class="Ring (strict)"("Visible"=TRUE) -> ()  [unwired: 2 in, 2 out]
                n184 = property on="Test Slider" class="Slide (strict)"("Visible"=FALSE) -> ()  [unwired: 2 in, 2 out]
              }
              frame "White Balance  **" {
                n185 = Index Array(array=w333, index=1) -> (element=w334:cluster{string[]})
                n186 = call <vilib>:"NT Read String.vi"("Name"=w336) -> ("String"=w335:string)  [unwired: 9 in, 1 out]
                n187 = Unbundle(w334) -> (w331:string[])
                n188 = Match First String(2:w331, 3:w335) -> (0:w330:i32)  [unwired: 1 out]
                n189 = property on="Test Ring" class="Ring (strict)"("Value"=w330, "Strings []"=w331) -> ()  [unwired: 2 in, 2 out]
                n190 = property on="Test Ring" class="Ring (strict)"("Visible"=TRUE) -> ()  [unwired: 2 in, 2 out]
                n191 = property on="Test Slider" class="Slide (strict)"("Visible"=FALSE) -> ()  [unwired: 2 in, 2 out]
              }
              frame "Exposure  **" {
                n192 = Index Array(array=w342, index=2) -> (element=w343:cluster{string[]})
                n193 = call <vilib>:"NT Read String.vi"("Name"=w345) -> ("String"=w344:string)  [unwired: 9 in, 1 out]
                n194 = Unbundle(w343) -> (w339:string[])
                n195 = Match First String(2:w339, 3:w344) -> (0:w340:i32)  [unwired: 1 out]
                n196 = property on="Test Ring" class="Ring (strict)"("Value"=w340, "Strings []"=w339) -> ()  [unwired: 2 in, 2 out]
                n197 = property on="Test Ring" class="Ring (strict)"("Visible"=TRUE) -> ()  [unwired: 2 in, 2 out]
                n198 = property on="Test Slider" class="Slide (strict)"("Visible"=FALSE) -> ()  [unwired: 2 in, 2 out]
              }
              frame "Exposure Priority  **" {
                n199 = Index Array(array=w351, index=3) -> (element=w352:cluster{string[]})
                n200 = call <vilib>:"NT Read String.vi"("Name"=w354) -> ("String"=w353:string)  [unwired: 9 in, 1 out]
                n201 = Unbundle(w352) -> (w348:string[])
                n202 = Match First String(2:w348, 3:w353) -> (0:w349:i32)  [unwired: 1 out]
                n203 = property on="Test Ring" class="Ring (strict)"("Value"=w349, "Strings []"=w348) -> ()  [unwired: 2 in, 2 out]
                n204 = property on="Test Ring" class="Ring (strict)"("Visible"=TRUE) -> ()  [unwired: 2 in, 2 out]
                n205 = property on="Test Slider" class="Slide (strict)"("Visible"=FALSE) -> ()  [unwired: 2 in, 2 out]
              }
              frame "Color Enable  **" {
                n206 = Index Array(array=w360, index=4) -> (element=w361:cluster{string[]})
                n207 = call <vilib>:"NT Read String.vi"("Name"=w363) -> ("String"=w362:string)  [unwired: 9 in, 1 out]
                n208 = Unbundle(w361) -> (w357:string[])
                n209 = Match First String(2:w357, 3:w362) -> (0:w358:i32)  [unwired: 1 out]
                n210 = property on="Test Ring" class="Ring (strict)"("Value"=w358, "Strings []"=w357) -> ()  [unwired: 2 in, 2 out]
                n211 = property on="Test Ring" class="Ring (strict)"("Visible"=TRUE) -> ()  [unwired: 2 in, 2 out]
                n212 = property on="Test Slider" class="Slide (strict)"("Visible"=FALSE) -> ()  [unwired: 2 in, 2 out]
              }
              frame Default {
                n213 = property on="Test Ring" class="Ring (strict)"("Visible"=FALSE) -> ()  [unwired: 2 in, 2 out]
                n214 = property on="Test Slider" class="Slide (strict)"("Visible"=FALSE) -> ()  [unwired: 2 in, 2 out]
              }
              frame "Brightness  **", "Color Level  **", "Compression  **", "FPS  **", "Sharpness  **" {
                n215 = call <vilib>:"NT Read Number.vi"("Name"=w369) -> ("Numeric"=w368:dbl)  [unwired: 9 in, 1 out]
                n216 = local write "Test Slider"(w368) -> ()
                n217 = property on="Test Slider" class="Slide (strict)"("Visible"=TRUE, "Scale.Maximum"=100.0 ("Scale.Range:Maximum")) -> ()  [unwired: 2 in, 2 out]
                n218 = property on="Test Ring" class="Ring (strict)"("Visible"=FALSE) -> ()  [unwired: 2 in, 2 out]
              }
            }
          }
        }
        n219 = property on="Progress" class="Clust (strict)"("Visible"=FALSE) -> ()  [unwired: 2 in, 2 out]
      }
      event "Test Name": Mouse Enter {
        # "Populate the ring with the list of tests"
        n220 = event-data() -> ()  [unwired: 1 in, 1 out]
        n221 = call <vilib>:"NT Read String Array.vi"("Name"="/TestMode/TestList") -> ("String Array"=w378:string[])  [unwired: 9 in, 1 out]
        n222 = Build Array (concatenate)("Select the test to run...", w378) -> (w377:string[])
        n223 = property on="Test Name" class="Ring (strict)"("Strings []"=w377) -> ()  [unwired: 2 in, 2 out]
      }
      event "Test Name": Value Change {
        w381 = FALSE ("Visible")
        # "Tell the robot the test name to run"
        n224 = event-data() -> ("NewVal"=w385:u16)  [unwired: 1 in]
        n225 = property on="Test Name" class="Ring (strict)"() -> ("Strings []"=w386:string[])  [unwired: 2 in, 2 out]
        n226 = local write "Progress"(T4 {"Test Progress"=0, "Test Progress Text"=""} ("Progress")) -> ()
        n227 = Index Array(array=w386, index=w385) -> (element=w384:string)
        n228 = call <vilib>:"NT Write String.vi"("String"=w384, "Name"="/TestMode/TestName") -> ()  [unwired: 9 in, 1 out]
        n229 = property on="Progress" class="Clust (strict)"("Visible"=TRUE) -> ()  [unwired: 2 in, 2 out]
        n230 = property on="Motor" class="Clust (strict)"("Visible"=w381) -> ()  [unwired: 2 in, 2 out]
        n231 = property on="Test Slider" class="Slide (strict)"("Visible"=w381) -> ()  [unwired: 2 in, 2 out]
        n232 = property on="On/Off" class="Bool (strict)"("Visible"=w381) -> ()  [unwired: 2 in, 2 out]
        n233 = property on="Rev/Fwd" class="Clust (strict)"("Visible"=w381) -> ()  [unwired: 2 in, 2 out]
        n234 = property on="Test Ring" class="Ring (strict)"("Visible"=w381) -> ()  [unwired: 2 in, 2 out]
      }
      event "Select Auto": Mouse Enter {
        # "Populate the combo box with the list of autonomous options"
        n235 = event-data() -> ()  [unwired: 1 in, 1 out]
        n236 = call <vilib>:"NT Read String Array.vi"("Name"="Auto List") -> ("String Array"=w388:string[])  [unwired: 9 in, 1 out]
        n237 = property on="Select Auto" class="CmbBox"("Strings[]"=w388) -> ()  [unwired: 2 in, 2 out]
      }
      event "Select Auto": Value Change {
        # "User modified the Auto Selection. Write to NT variable so robot knows."
        n238 = event-data() -> ("NewVal"=w392:string)  [unwired: 1 in]
        n239 = call <vilib>:"NT Write String.vi"("String"=w392, "Name"="Auto Selector") -> ()  [unwired: 9 in, 1 out]
      }
      event "Command Selection": Value Change {
        # "Get the params and show in table"
        n240 = event-data() -> ("NewVal"=w399:i32)  [unwired: 1 in]
        n241 = property on="Command Selection" class="MCListbox (strict)"() -> ("ItemNames"=w397:string[][])  [unwired: 2 in, 2 out]
        n242 = call <vilib>:"WPI_DashboardUpdate Command Params.vi"("NewVal"=w399, "Commands"=w397, "Param Tbl"=w398) -> ()  [unwired: 8 in, 1 out]
      }
      event "Execute Command": Value Change {
        # "Started one, Unique ID holds\nresponse"
        n243 = event-data() -> ()  [unwired: 1 in, 1 out]
        n244 = property on="Command Selection" class="MCListbox (strict)"() -> ("ItemNames"=w411:string[][])  [unwired: 2 in, 2 out]
        n245 = Index Array(array=w411, index (row)="Command Selection", index (col)=0) -> (element=w409:string)
        n246 = call <vilib>:"Invoke Commands.vi"("Command Params"="Command Params", "Function Name"=w409) -> ("Params"=w405:u8, "Started"=w404:bool)  [unwired: 7 in, 1 out]
        n247 = Array Subset(array="Command Params", length (row)=w405) -> (w406:string[][])  [unwired: 3 in]
        n248 = Select(t="Executing" ("Cmd Status"), s=w404, f="" ("Cmd Status")) -> (s? t:f=→"Cmd Status":string)
      }
      event "Command Selection": Double Click {
        n249 = event-data() -> ("Row"=w421:i32)  [unwired: 1 in]
        n250 = property on="Command Selection" class="MCListbox (strict)"() -> ("ItemNames"=w424:string[][])  [unwired: 2 in, 2 out]
        n251 = local read "Command Params"() -> (w419:string[][])
        n252 = Index Array(array=w424, index (row)=w421, index (col)=0) -> (element=w422:string)
        n253 = call <vilib>:"Invoke Commands.vi"("Command Params"=w419, "Function Name"=w422) -> ("Params"=w418:u8, "Started"=w413:bool)  [unwired: 7 in, 1 out]
        n254 = Array Subset(array=w419, length (row)=w418) -> (w417:string[][])  [unwired: 3 in]
        n255 = Select(t="Executing" ("Cmd Status"), s=w413, f="" ("Cmd Status")) -> (s? t:f=w414:string)
        n256 = local write "Cmd Status"(w414) -> ()
      }
      event "CheckList": Double Click {
        # "Shift clears all"
        # "Update symbols on the listbox"
        n257 = event-data() -> ("PlatMods.Shift"=w427:bool, "Row"=w429:i32)  [unwired: 1 in]
        n258 = case shown="True" w427 {
          tunnel: w429 -> [w433 _]
          tunnel: 1 -> [w432 _]
          frame False {
            n259 = property on="CheckList" class="LstBox (strict)"() -> ("Item Symbols"=w431:i32[])  [unwired: 2 in, 2 out]
            n260 = Replace Array Subset(array=w431, new element=w432, index=w433) -> (w430:i32[])
            n261 = property on="CheckList" class="LstBox (strict)"("Item Symbols"=w430) -> ()  [unwired: 2 in, 2 out]
          }
          frame True {
            w434 = 0 ("Top Row")
            n262 = property on="CheckList" class="LstBox (strict)"() -> ("Number of Rows"=w436:u32)  [unwired: 2 in, 2 out]
            n263 = Initialize Array(0, w436) -> (w435:i32[])
            n264 = property on="CheckList" class="LstBox (strict)"("Top Row"=w434, "Value"=w434, "Item Symbols"=w435) -> ()  [unwired: 2 in, 2 out]
          }
        }
      }
      event "CheckList": Key Down {
        # "Update symbols on the listbox\nLeft and right keys check and uncheck"
        n265 = event-data() -> ("VKey"=w441:T16)  [unwired: 1 in]
        n266 = case shown="\"Left\", \"Right\"" w441 {
          selector: w441 -> [w446 _]
          tunnel: eventvkey."Left" ("VKey") -> [w444 _]
          frame "Left", "Right" {
            n267 = Equal?(x=w444, y=w446) -> (x = y?=w445:bool)
            n268 = Select(t=0, s=w445, f=1) -> (s? t:f=w447:i32)
            n269 = property on="CheckList" class="LstBox (strict)"() -> ("Item Symbols"=w450:i32[])  [unwired: 2 in, 2 out]
            n270 = Replace Array Subset(array=w450, new element=w447, index="CheckList") -> (w449:i32[])
            n271 = property on="CheckList" class="LstBox (strict)"("Item Symbols"=w449) -> ()  [unwired: 2 in, 2 out]
          }
          frame Default {
          }
        }
      }
      event "DB Camera Config": Value Change {
        # "Show or hide the cluster of controls, store in ini file"
        n272 = event-data() -> ("NewVal"=w455:bool)  [unwired: 1 in]
        n273 = case shown="False" w455 {
          tunnel: w454 -> [w464 _]
          tunnel: [w457 w475] -> w453
          tunnel: w452 -> [w456 w475]
          frame False {
            w471 = "Camera"
            w474 = FALSE ("Visible")
            n274 = local read "Camera Settings"() -> (w463:T2)
            n275 = Index Array(array=w464) -> (element=w467:cluster{string[]})  [unwired: 1 in]
            n276 = Unbundle(w463) -> ("Frame Rate"=w462:i32, "Compression"=w461:i32, "Size"=w465:u16)
            n277 = Unbundle(w467) -> (w466:string[])
            n278 = Index Array(array=w466, index=w465) -> (element=w460:string)
            n279 = call-poly <vilib>:"Write Key.vi"("section"=w471, "value"=w460, "key"="Size", "refnum"=w456) -> ("refnum out"=w473:T14)  [unwired: 2 in, 5 out]
            n280 = call-poly <vilib>:"Write Key.vi"("section"=w471, "value"=w462, "key"="FrameRate", "refnum"=w473) -> ("refnum out"=w472:T14)  [unwired: 1 in, 6 out]
            n281 = property on="Camera Settings" class="Clust (strict)"("Visible"=w474) -> ()  [unwired: 2 in, 2 out]
            n282 = local write "DB Camera Config"(w474) -> ()
            n283 = call-poly <vilib>:"Write Key.vi"("section"=w471, "value"=w461, "key"="Compression", "refnum"=w472) -> ("refnum out"=w458:T14)  [unwired: 1 in, 6 out]
            n284 = call <vilib>:"Close Config Data.vi"("refnum"=w458) -> ("file path"=w459:path)  [unwired: 2 in, 8 out]
            n285 = call <vilib>:"Open Config Data.vi"("configuration file path"=w459) -> ("refnum"=w457:T14)  [unwired: 8 in, 2 out]
          }
          frame True {
            n286 = property on="Camera Settings" class="Clust (strict)"("Visible"=TRUE) -> ()  [unwired: 2 in, 2 out]
          }
        }
      }
      event "Camera Settings": Value Change {
        # "Update summary string when any elements of DB camera change"
        n287 = event-data() -> ("NewVal"=w489:T2)  [unwired: 1 in]
        n288 = Index Array(array=w485) -> (element=w484:cluster{string[]})  [unwired: 1 in]
        n289 = Unbundle(w489) -> ("Frame Rate"=w480:i32, "Compression"=w479:i32, "Size"=w482:u16)
        n290 = Unbundle(w484) -> (w483:string[])
        n291 = Index Array(array=w483, index=w482) -> (element=w481:string)
        n292 = Format Into String(format string="%s   %dfps   %d%%", w481, w480, w479) -> (resulting string=w486:string)  [unwired: 2 in, 1 out]
        n293 = Build Array(w486) -> (w487:string[])
        n294 = property on="DB Camera Config" class="Bool (strict)"("Strings [4]"=w487) -> ()  [unwired: 2 in, 2 out]
      }
      event "Motor.Enable": Value Change {
        # "When the test mode otor enable helper is set, update that\ntree row item's value"
        n295 = event-data() -> ("NewVal"=w496:bool)  [unwired: 1 in]
        n296 = Unbundle("Motor") -> ("Value"=w495:dbl)  [unwired: 1 out]
        n297 = Select(t=w495, s=w496, f=0.0) -> (s? t:f=w493:dbl)
        n298 = call <vilib>:"NT Write Number.vi"("Numeric"=w493, "Name"=w492) -> ()  [unwired: 9 in, 1 out]
      }
      event "Test Slider": Value Change {
        # "When the test mode slider helper is set, update that\ntree row item's value"
        n299 = event-data() -> ("NewVal"=w500:dbl)  [unwired: 1 in]
        n300 = call <vilib>:"NT Write Number.vi"("Numeric"=w500, "Name"=w501) -> ()  [unwired: 9 in, 1 out]
      }
      event "On/Off": Value Change {
        # "When the test mode on/off helper value is set, update that\ntree row item's value"
        n301 = event-data() -> ("NewVal"=w506:bool)  [unwired: 1 in]
        n302 = Boolean To (0,1)(Boolean=w506) -> (0, 1=w505:i16)
        n303 = call <vilib>:"NT Write Number.vi"("Numeric"=w505, "Name"=w504) -> ()  [unwired: 9 in, 1 out]
      }
      event "Rev/Fwd": Value Change {
        # "When the test mode helper value for relays is set, update that\ntree row item's value"
        n304 = event-data() -> ("NewVal.Forward"=w515:bool, "NewVal.Reverse"=w514:bool)  [unwired: 1 in]
        n305 = Boolean To (0,1)(Boolean=w515) -> (0, 1=w511:i16)
        n306 = Boolean To (0,1)(Boolean=w514) -> (0, 1=w513:i16)
        n307 = Negate(x=w513) -> (-x=w512:i16)
        n308 = Add(x=w511, y=w512) -> (x+y=w510:i16)
        n309 = call <vilib>:"NT Write Number.vi"("Numeric"=w510, "Name"=w509) -> ()  [unwired: 9 in, 1 out]
      }
      event "Test Ring": Value Change {
        # "When a test mode helper value is selected from the ring,\nset the tree item's variable to the string value"
        n310 = event-data() -> ("NewVal"=w520:u16)  [unwired: 1 in]
        n311 = property on="Test Ring" class="Ring (strict)"() -> ("Strings []"=w521:string[])  [unwired: 2 in, 2 out]
        n312 = Index Array(array=w521, index=w520) -> (element=w519:string)
        n313 = call <vilib>:"NT Write String.vi"("String"=w519, "Name"=w518) -> ()  [unwired: 9 in, 1 out]
      }
      event "Rec Mode": Value Change {
        # "Update globals for recording mode and path to read log from.\nClear when logging and let NetworkTables set path for vision to\nuse."
        n314 = event-data() -> ("NewVal"=w533:enum32{"Stop", "Record", "Playback"})  [unwired: 1 in]
        n315 = global write "WPI_DashboardLogging Global.vi" "Logging Filename"(path "") -> ()
        n316 = global write "WPI_DashboardLogging Global.vi" "Recording"(w533) -> ()
        n317 = case shown="\"Playback\"" w533 {
          tunnel: w532 -> [_ w535 w544]
          tunnel: [_ _ w543] -> w529
          tunnel: [_ _ w542] -> _
          tunnel: w527 -> [_ _ w540]
          tunnel: cluster{i32, i32} {-250, 170} -> [_ _ w539]
          tunnel: [_ _ T17 {"Image Size"=TRUE, "Image Type"=TRUE, "Pixel Value"=TRUE, "ROI Information"=TRUE, "Zoom Factor"=FALSE} ("Image Information Shown:All Elements")] -> w525
          tunnel: [_ _ TRUE ("Zoom Factor")] -> w524
          tunnel: w523 -> [_ _ w536]
          frame Default {
          }
          frame "Stop", "Record" {
            # "Place Window too"
            n318 = invoke class="VI" method="FP.Close"(reference=w535) -> (reference out=w534:refnum<vi>)  [unwired: 2 in, 2 out]
            n319 = invoke class="VI" method="Abort VI"(reference=w534) -> ()  [unwired: 2 in, 3 out]
          }
          frame "Playback" {
            n320 = call "Open Playback Panel.vi"("Offset"=w539, "DB VI Ref"=w540, "Playback in"=w544) -> ("Playback out"=w541:refnum<vi>)  [unwired: 8 in]
            n321 = register-events(w541, w536) -> (reference out=w543:refnum<event-registration>, error out=w542:errorcluster)  [unwired: 2 in]
          }
        }
        n322 = property on="Camera Image" class="ImageControl"("Image Information Shown"=w525, "Image Information Visible"=w524) -> ()  [unwired: 2 in, 2 out]
        n323 = call <vilib>:"WPI_DashboardNT Log FieldName Cache.vi"("Operation"=enum16{"Lookup/Add", "Index", "Clear"}."Clear") -> ()  [unwired: 8 in, 3 out]
      }
      event Panel Close {
        w546 = enum32{"Stop", "Record", "Playback"}."Stop" ("Rec Mode")
        # "Playback window has been closed, abort"
        n324 = event-data() -> ()  [unwired: 1 in, 4 out]
        n325 = local write "Rec Mode"(w546) -> ()
        n326 = global write "WPI_DashboardLogging Global.vi" "Recording"(w546) -> ()
      }
      event Panel Close {
        # "Abort playback window and ourself"
        n327 = event-data() -> ()  [unwired: 1 in, 4 out]
        n328 = invoke class="VI" method="FP.Close"(reference=w552) -> (reference out=w551:refnum<vi>)  [unwired: 2 in, 2 out]
        n329 = invoke class="VI" method="Abort VI"(reference=w551) -> (error out=w550:errorcluster)  [unwired: 2 in, 2 out]
        n330 = invoke class="VI" method="Abort VI"(error in=w550) -> ()  [unwired: 2 in, 3 out]
      }
      event User Event {
        n331 = event-data() -> ("IDs"=w560:cluster{"RPC field ID":u16, "Unique ID":u16}, "String"=w559:string)  [unwired: 1 in]
        n332 = Bundle("IDs"=w560, "String"=w559) -> (w558:T6)  [unwired: 1 in]
        n333 = call <vilib>:"Retrieve RPC Response.vi"("RPC Response"=w558) -> ("Output"=w555:string[][])  [unwired: 10 in]
        n334 = Build Array (concatenate)(w553, w555) -> (w554:string[][])
        n335 = local write "Command Params"(w554) -> ()
        n336 = local write "Cmd Status"("" ("Cmd Status")) -> ()
      }
      event "Vision": Value Change {
        # "Enable/Disable Compression slider.\nHW USB is hard-coded into the camera"
        n337 = event-data() -> ("NewVal"=w567:u16)  [unwired: 1 in]
        n338 = Equal?(x=w567, y=u32 2 ("milliseconds to wait")) -> (x = y?=w565:bool)
        n339 = Select(t=T18."Disabled and Grayed Out" ("Disabled"), s=w565, f=T18."Enabled" ("Disabled")) -> (s? t:f=w562:T18)
        n340 = property on="Compression" class="Slide (strict)"("DisabledEnum"=w562) -> ()  [unwired: 2 in, 2 out]
      }
      event "Tree": Double Click {
        n341 = event-data() -> ("PlatMods"=w572:T21, "Tag"=w571:string)  [unwired: 1 in]
        n342 = Unbundle(w572) -> ("Shift"=w570:bool)  [unwired: 4 out]
        n343 = Not(x=w570) -> (.not. x?=w569:bool)
        n344 = call <vilib>:"NT Update Persistence.vi"("Persistence"=w569, "Name"=w571) -> ()  [unwired: 9 in, 1 out]
      }
    }
  }
  n345 = while {
    tunnel: w50 -> [w576]
    i -> [w579]
    stop <- FALSE stop-if-true
    n346 = Wait (ms)(milliseconds to wait=u32 100) -> ()  [unwired: 1 out]
    n347 = case shown="\"Playback\"" "Rec Mode" {
      tunnel: w579 -> [_ _ w594]
      tunnel: [u32 2829099 ("Base Color") u32 11141120 ("Target Color") w583] -> w575
      frame "Stop", Default {
        # "Reset the color, extra updates don't cost much"
      }
      frame "Record" {
      }
      frame "Playback" {
        # "Playback"
        n348 = Quotient & Remainder(x=w594, y=u32 50 ("milliseconds to wait")) -> (x-y*floor(x/y)=w590:u32)  [unwired: 1 out]
        n349 = Divide(x=w590, y=u32 50 ("milliseconds to wait")) -> (x/y=w587:dbl)
        n350 = Multiply(x=6.283185307179586, y=w587) -> (x*y=w592:dbl)
        n351 = Sine(x=w592) -> (sin(x)=w591:dbl)
        n352 = Absolute Value(x=w591) -> (abs(x)=w584:dbl)
        n353 = call "Interpolate RGB Color.vi"("Proportion"=w584, "Target Color"=u32 30976, "Base Color"=u32 2829099) -> ("Result Color"=w583:u32)  [unwired: 8 in]
      }
    }
    n354 = property class="Pane"(reference=w576, "PaneColor"=w575) -> ()  [unwired: 1 in, 2 out]
  }
  n355 = call <vilib>:"System Exec.vi"("wait until completion? (T)"=FALSE, "working directory"=path "C:/Users/Rick/Desktop/Dashboard-2016", "command line"="py main.py") -> ()  [unwired: 5 in, 4 out]
  n356 = local write "Dashboard Tab"(T1."Drive" ("Dashboard Tab")) -> ()
  n357 = property on="On/Off" class="Bool (strict)"("Visible"=w18) -> ()  [unwired: 2 in, 2 out]
  n358 = property on="Motor" class="Clust (strict)"("Visible"=w18) -> ()  [unwired: 2 in, 2 out]
  n359 = property on="Progress" class="Clust (strict)"("Visible"=w18) -> ()  [unwired: 2 in, 2 out]
  n360 = property on="Test Ring" class="Ring (strict)"("Visible"=w18) -> ()  [unwired: 2 in, 2 out]
  n361 = property on="Rev/Fwd" class="Clust (strict)"("Visible"=w18) -> ()  [unwired: 2 in, 2 out]
  n362 = property on="Camera Settings" class="Clust (strict)"("Visible"=w18) -> ()  [unwired: 2 in, 2 out]
  n363 = while {
    tunnel: u16 1741 ("timeout ms (25000)") -> [w596]
    stop <- FALSE stop-if-true
    n364 = TCP Create Listener(10:w596) -> (0:w595:errorcluster, 3:w597:refnum<k5>)  [unwired: 4 in, 1 out]
    n365 = case shown="No Error" w595 {
      selector: w595 -> [w599 _]
      tunnel: w597 -> [w600 _]
      frame No Error {
        n366 = while {
          tunnel: w600 -> [w603]
          tunnel: w599 -> [w602]
          stop <- FALSE stop-if-true
          n367 = TCP Wait On Listener(8:w602, 11:w603) -> (0:w604:errorcluster, 4:w605:refnum<k5>)  [unwired: 2 in, 3 out]
          n368 = local write "TCP"(w605) -> ()
          n369 = case shown="No Error" w604 {
            frame No Error {
            }
            frame Error {
              n370 = Wait (ms)(milliseconds to wait=u32 1000) -> ()  [unwired: 1 out]
            }
          }
        }
      }
      frame Error {
        n371 = Wait (ms)(milliseconds to wait=u32 1000) -> ()  [unwired: 1 out]
      }
    }
  }
  n372 = local write "DB Camera Config"(w18) -> ()
  n373 = local write "Command Params"(string[][] [] ("Command Params")) -> ()
  n374 = global write "WPI_DashboardLogging Global.vi" "Recording"(w44) -> ()
  n375 = local write "Command Selection"(u16 0 ("milliseconds to wait")) -> ()
  n376 = local write "Rec Mode"(w44) -> ()
